vi "删除大于零.vi"(2 "数组－数值 2":dbl[](array[numeric]), 3 "数组－数值":dbl[](array[numeric])) -> (0 "第二列":dbl[](array[numeric]), 1 "第一列":dbl[](array[numeric]))   [LabVIEW 2016]
panel:
  in  "数组 4":dbl[](array[numeric])
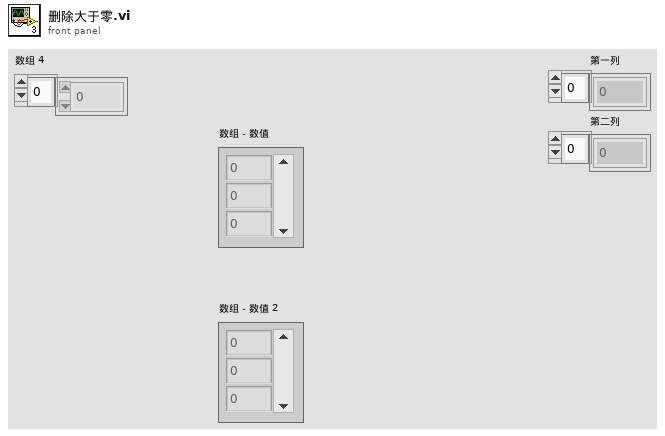
[diagram p1: front panel]
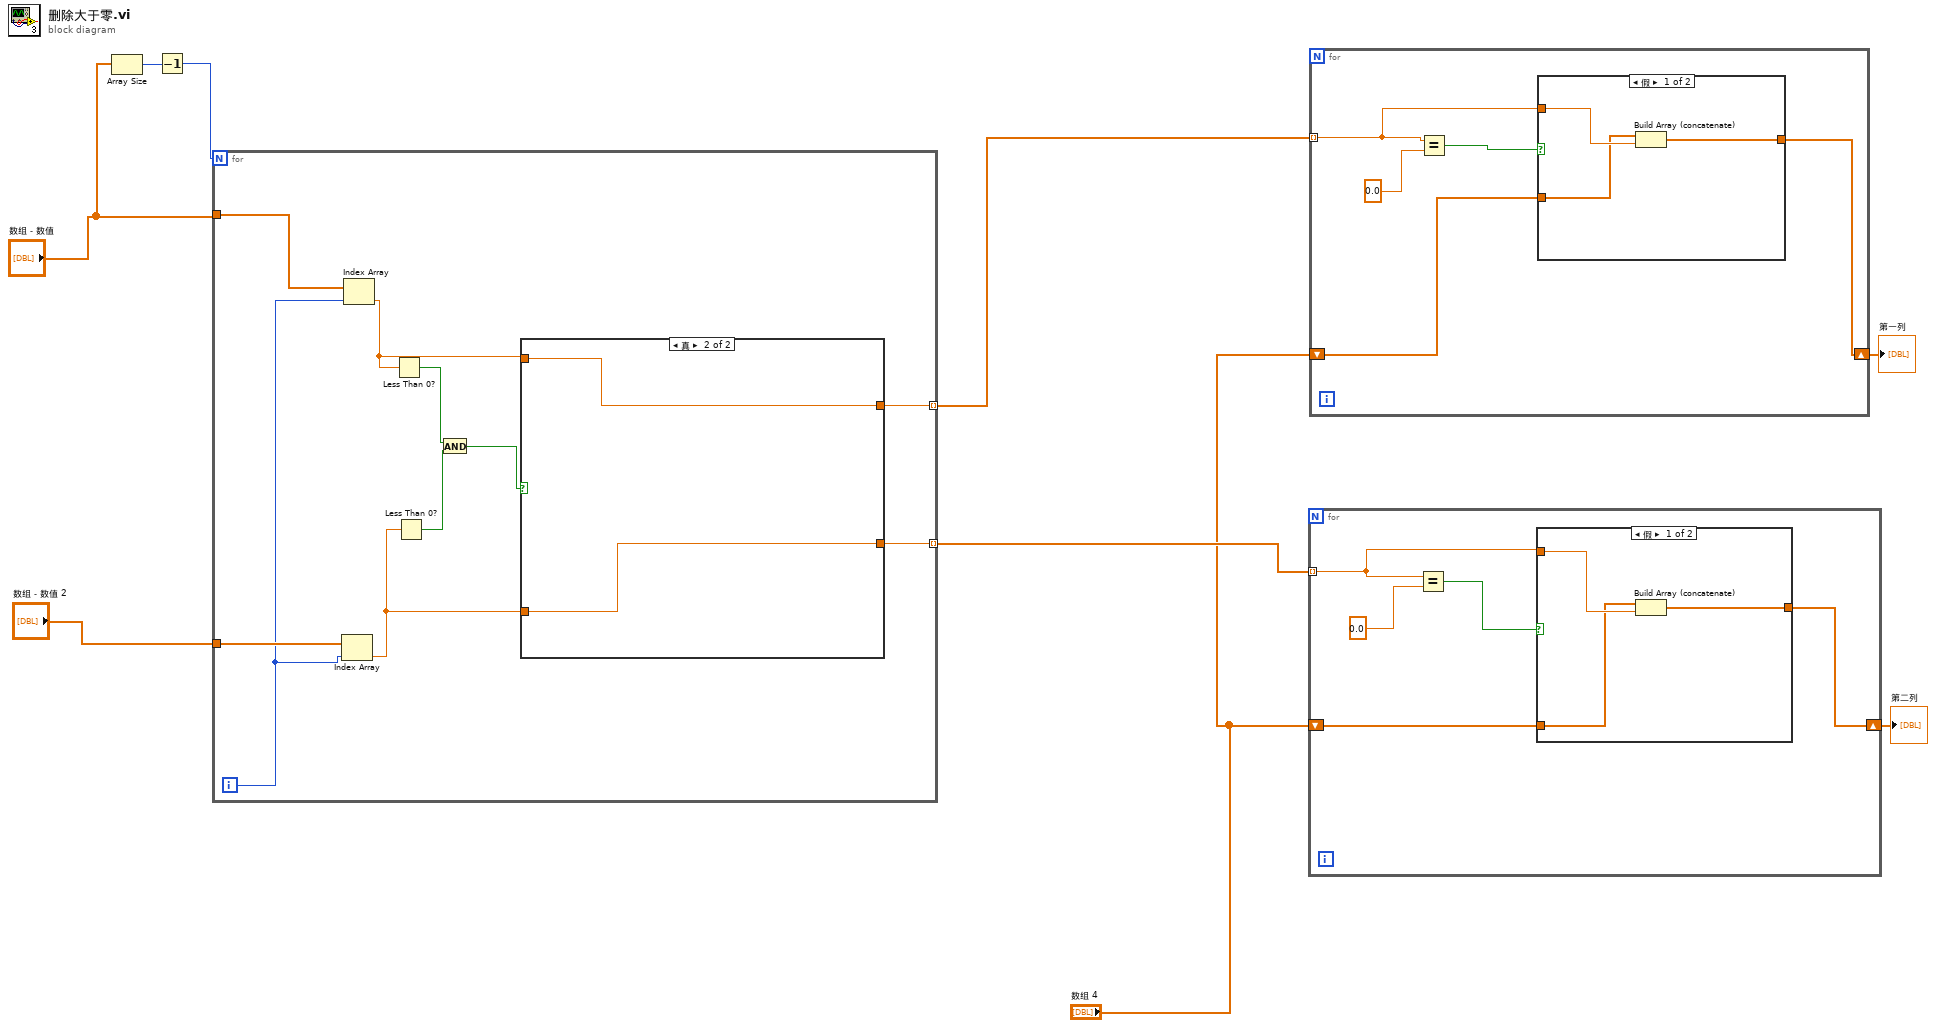
[diagram p0: block diagram]
diagram:
  n1 = Array Size(array="数组－数值") -> (size(s)=w9:i32)
  n2 = Decrement(x=w9) -> (x-1=w8:i32)
  n3 = for {
    N: w8 -> [_]
    tunnel: "数组－数值" -> [w19]
    tunnel: "数组－数值 2" -> [w18]
    tunnel: [w11] -> w5 mode=indexing
    tunnel: [w10] -> w4 mode=indexing
    i -> [w17]
    n4 = Index Array(array=w18, index=w17) -> (element=w12:dbl)
    n5 = Index Array(array=w19, index=w17) -> (element=w13:dbl)
    n6 = Less Than 0?(x=w13) -> (x < 0?=w16:bool)
    n7 = Less Than 0?(x=w12) -> (x < 0?=w15:bool)
    n8 = And(x=w16, y=w15) -> (x .and. y?=w14:bool)
    n9 = case shown="真" w14 {
      tunnel: w13 -> [_ w21]
      tunnel: w12 -> [_ w20]
      tunnel: [_ w21] -> w11
      tunnel: [_ w20] -> w10
      frame False {
      }
      frame True {
      }
    }
  }
  n10 = for {
    tunnel: w4 -> [w24] mode=indexing
    shift-right: [w22] -> w1
    shift-left: "数组 4" -> [w23]
    n11 = Equal?(x=w24, y=0.0) -> (x = y?=w25:bool)
    n12 = case shown="假" w25 {
      tunnel: w24 -> [w29 _]
      tunnel: w23 -> [w28 w30]
      tunnel: [w27 w30] -> w22
      frame False {
        n13 = Build Array (concatenate)(w28, w29) -> (w27:dbl[])
      }
      frame True {
      }
    }
  }
  "第二列" <- w1
  n14 = for {
    tunnel: w5 -> [w33] mode=indexing
    shift-right: [w31] -> w2
    shift-left: "数组 4" -> [w32]
    n15 = Equal?(x=w33, y=0.0) -> (x = y?=w34:bool)
    n16 = case shown="假" w34 {
      tunnel: w33 -> [w38 _]
      tunnel: w32 -> [w37 w39]
      tunnel: [w36 w39] -> w31
      frame False {
        n17 = Build Array (concatenate)(w37, w38) -> (w36:dbl[])
      }
      frame True {
      }
    }
  }
  "第一列" <- w2
